vi "Profile Auton - Angle.vi"(8 "error in (no error)":errorcluster, 10 "Time (s)":dbl, 11 "Angle (degrees)":dbl) -> (0 "error out":errorcluster)   [LabVIEW 2017]
uses:
  <vilib>/Rock Robotics/WPI/ThirdParty/Sensors/navX/_TypeDefs/FRIC_navX_DeviceNumbersTypeDef.ctl
  Robot Global Data.vi
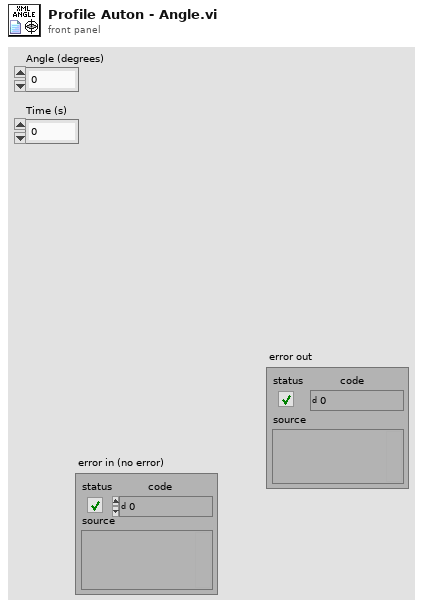
[diagram p1: front panel]
types:
  T1 = typedef "FRIC_navX_DeviceNumbersTypeDef.ctl" = enum16{"Dev0", "Dev1", "Dev2", "Dev3"}
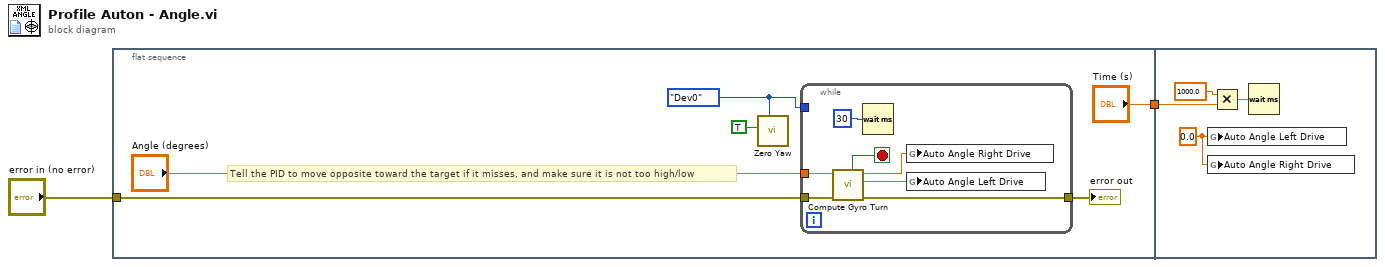
[diagram p0: block diagram]
diagram:
  n1 = flat-sequence {
    tunnel: ["Time (s)"] -> w2
    tunnel: "error in (no error)" -> [w5]
    tunnel: w2 -> [w17]
    frame #0 {
      w3 = FRIC_navX_DeviceNumbersTypeDef."Dev0" ("Device Number")
      # "Tell the PID to move opposite toward the target if it misses, and make sure it is not too high/low"
      n2 = call <vilib>:"Zero Yaw.vi"("Device Number"=w3, "Zero"=TRUE) -> ()  [unwired: 10 in]
      n3 = while {
        tunnel: [w13] -> w8
        tunnel: "Angle (degrees)" -> [w12]
        tunnel: w5 -> [w11]
        tunnel: w3 -> [_]
        stop <- w14 stop-if-true
        n4 = call "Compute Gyro Turn.vi"("error in (no error)"=w11, "Turn? Right Positive."=w12) -> ("error out"=w13:errorcluster, "Right Drive"=w10:dbl, "Left drive"=w9:dbl, "done"=w14:bool)  [unwired: 6 in]
        n5 = Wait (ms)(milliseconds to wait=u32 30) -> ()  [unwired: 1 out]
        n6 = global write "Robot Global Data.vi" "Auto Angle Right Drive"(w9) -> ()
        n7 = global write "Robot Global Data.vi" "Auto Angle Left Drive"(w10) -> ()
      }
      "error out" <- w8
    }
    frame #1 {
      w16 = 0.0
      n8 = global write "Robot Global Data.vi" "Auto Angle Left Drive"(w16) -> ()
      n9 = global write "Robot Global Data.vi" "Auto Angle Right Drive"(w16) -> ()
      n10 = Multiply(x=1000.0, y=w17) -> (x*y=w19:dbl)
      n11 = Wait (ms)(milliseconds to wait=w19) -> ()  [unwired: 1 out]
    }
  }
